vi "_SendCommand.vi"(8 "error in":errorcluster, 10 "Command":string, 11 "Instrument Channel":string="GPIB/0:4,0") -> (0 "error out":errorcluster, 3 "Instrument Channel out":string="GPIB/0:4,0")   [LabVIEW 2020]
doc: "Send command string to instrument channel."
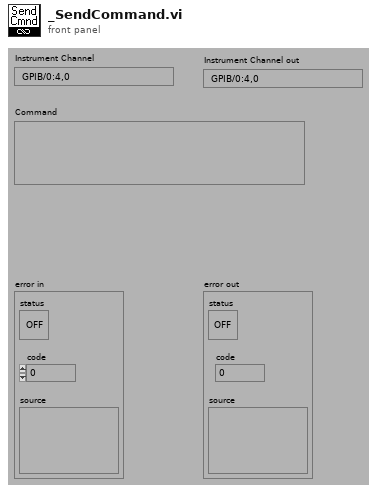
[diagram p1: front panel]
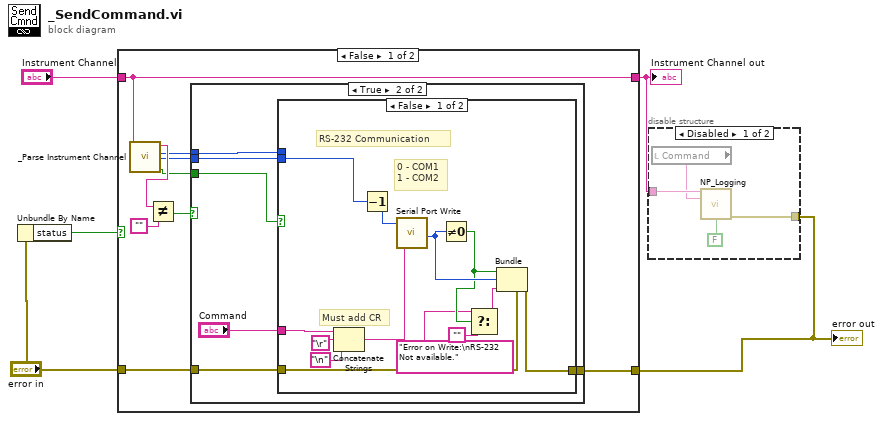
[diagram p0: block diagram]
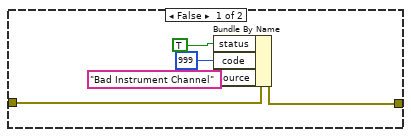
[diagram p3: hidden frame]
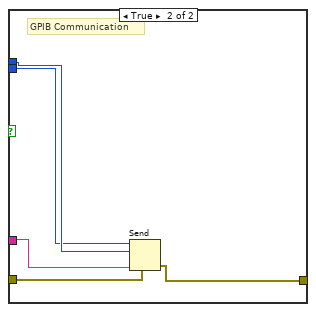
[diagram p4: hidden frame]
diagram:
  n1 = Unbundle By Name("error in") -> ("status"=w4:bool)
  n2 = case shown="False" w4 {
    tunnel: "error in" -> [w14 w44]
    tunnel: "Instrument Channel" -> [w10 w45]
    tunnel: [w10 w45] -> w2
    tunnel: [w9 w44] -> w1
    frame False {
      n3 = call "_Parse Instrument Channel.vi"("Instrument Channel"=w10) -> ("T - GPIB, F - RS232"=w7:bool, "Hardware Address"=w6:i32, "Instrument Address"=w8:i16, "Instrument Channel out"=w11:string)  [unwired: 6 in, 1 out]
      n4 = Not Equal?(x=w11, y="") -> (x != y?=w12:bool)
      n5 = case shown="True" w12 {
        tunnel: w14 -> [w16 w24]
        tunnel: [w15 w23] -> w9
        tunnel: w8 -> [_ w22]
        tunnel: w7 -> [_ w21]
        tunnel: w6 -> [_ w20]
        frame False {
          n6 = Bundle By Name(cluster=w16, "status"=TRUE, "code"=999, "source"="Bad Instrument Channel") -> (w15:errorcluster)
        }
        frame True {
          n7 = case shown="False" w21 {
            tunnel: "Command" -> [w38 w43]
            tunnel: w24 -> [w37 w42]
            tunnel: [w36 w41] -> w23
            tunnel: w22 -> [_ w40]
            tunnel: w20 -> [w26 w39]
            frame False {
              # "0 - COM1\n1 - COM2"
              # "Must add CR"
              # "RS-232 Communication"
              n8 = Concatenate Strings(w38, "\r", "\n") -> (w31:string)
              n9 = Decrement(x=w26) -> (x-1=w27:i32)
              n10 = call "Serial Port Write.vi"("string to write"=w31, "port number"=w27) -> ("error code"=w35:i32)
              n11 = Not Equal To 0?(x=w35) -> (x != 0?=w34:bool)
              n12 = Select(t="Error on Write:\nRS-232 Not available.", s=w34, f="") -> (s? t:f=w33:string)
              n13 = Bundle(cluster=w37, "status"=w34, "code"=w35, "source"=w33) -> (w36:errorcluster)
            }
            frame True {
              # "GPIB Communication"
              n14 = Send(0:w39, 2:w40, 4:w42, 5:w43) -> (8:w41:errorcluster)  [unwired: 1 in, 2 out]
            }
          }
        }
      }
    }
    frame True {
      # "Error Status is True"
    }
  }
  "Instrument Channel out" <- w2
  "error out" <- w1
  n15 = disable-structure shown="Disabled" {
    disable-tunnel: w2 -> [w49 _]
    disable-tunnel: w1 -> [w48 _]
    frame Disabled {
      n16 = local read "Command"() -> (w47:string)
      n17 = call "NP_Logging.vi"("Instrument Channel"=w49, "String 1 {Write} (in)"=w47, "error in (no error)"=w48, "String 2 Enable (T)"=FALSE) -> ()  [unwired: 8 in, 4 out]
    }
    frame Enabled {
    }
  }
